vi "libssh2_knownhost_get - invalid known hosts collection - returns invalid host.vi"() -> ()   [LabVIEW 2017, in "unit_tests.lvlib"]
uses:
  unit_tests.lvlib
  libssh2/Host Key Database Refnum.ctl
  libssh2/libssh2_init_default.vi
  libssh2/libssh2_session_init_ex.vi
  libssh2/libssh2.lvlib
  <vilib>/PNR/Transparent Assertions/Transparent Assertions/Transparent Assertions.lvlib
panel:
  out "error out":errorcluster
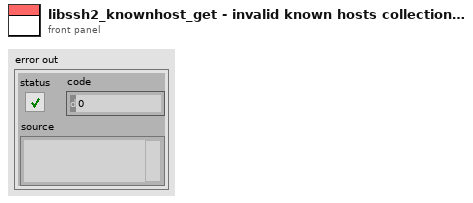
[diagram p1: front panel]
types:
  T1 = typedef "libssh2.lvlib/Session Refnum.ctl" = refnum<k1>
  T2 = typedef "libssh2.lvlib/Host Key Database Refnum.ctl" = refnum<k1>
  T3 = typedef "libssh2.lvlib/Host Key Refnum.ctl" = refnum<k1>
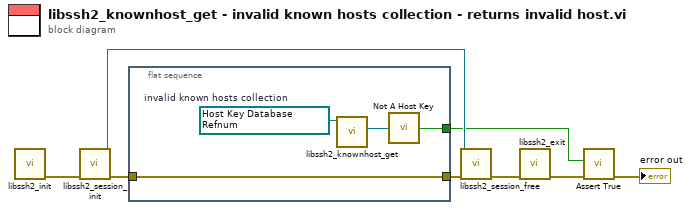
[diagram p0: block diagram]
diagram:
  n1 = call-poly "libssh2_init.vi"() -> ("error out"=w7:errorcluster)  [unwired: 11 in]
  n2 = call "libssh2_session_init.vi"("error in (no error)"=w7) -> ("error out"=w1:errorcluster, "session"=w4:T1)  [unwired: 9 in]
  n3 = flat-sequence {
    tunnel: [w12] -> w3
    tunnel: [w11] -> w2
    tunnel: w1 -> [w11]
    frame #0 {
      w10 = T2 refnum items=["host key database"]  # invalid known hosts collection
      n4 = call "libssh2_knownhost_get.vi"("host key database"=w10) -> ("host key"=w9:T3)  [unwired: 8 in, 2 out]
      n5 = call "Not A Host Key.vi"("host key"=w9) -> ("Not a Host Key?"=w12:bool)
    }
  }
  n6 = call "libssh2_session_free.vi"("error in (no error)"=w2, "session"=w4) -> ("error out"=w6:errorcluster)  [unwired: 9 in]
  n7 = call "libssh2_exit.vi"("error in (no error)"=w6) -> ("error out"=w5:errorcluster)  [unwired: 10 in]
  n8 = call <vilib>:"Assert True.vi"("error in (no error)"=w5, "Condition"=w3) -> ("error out"=→"error out":errorcluster)  [unwired: 9 in]
